vi "command data test.vi"() -> ()   [LabVIEW 2020]
panel:
  out "number":u32=24
  out "Array 2":string[](array[string])=["init\r\n", "runRange\r\n", "trackOn\r\n", "trackOff\r\n", "setLoad>1\r\n", "setMot>1\r\n", "setKp>1\r\n", "setKi>1\r\n", "setKd>1\r\n", "setR>1\r\n", "setG>1\r\n", "setB>1\r\n", "motOn\r\n", "motOff\r\n", "getVolts<1\r\n", "getBV<2\r\n", "getVal<1\r\n", "getKW<1\r\n", "getCarbon<1\r\n", "getAll<7\r\n", "getRes<1\r\n", "getDrop<1\r\n", "getCurrent<1\r\n", "off\r\n", "eoc\r\n"]
  out "Count":dbl=22.0
  in  "Array":string[](array[string])=["init", "runRange", "trackOn", "trackOff", "setLoad>1", "setMot>1", "setKp>1", "setKi>1", "setKd>1", "setR>1", "setG>1", "setB>1", "motOn", "motOff", "getVolts<1", "getBV<2", "getVal<1", "getKW<1", "getCarbon<1", "getAll<7", "getRes<1", "getDrop<1", "getCurrent<1", "off", "eoc"]
  in  "String":string="\"init\",\"runRange\", \"trackOn\",\"trackOff\",\n                    \"setLoad>1\",\"setMot>1\",\"setKp>1\",\"setKi>1\",\"setKd>1\",\"setR>1\",\"setG>1\",\"setB>1\",\n                    \"motOn\",\"motOff\",\n                    \"getVolts<1\", \"getBV<2\",\n                    \"getVal<1\",\"getKW<1\",\"getCarbon<1\",\"getAll<7\",\"getRes<1\",\"getDrop<1\",\"getCurrent<1\", \n                    \"off\",\"eoc\""
  out "read buffer":string="eoc\r\n"
  out "Device Name 2":string[](array[string])=["generator\r\n"]
  out "Num Dev 2":u32=1
  out "Device Address 2":refnum<visa-resource-name>[](array[refnum])=["ASRL28::INSTR"]
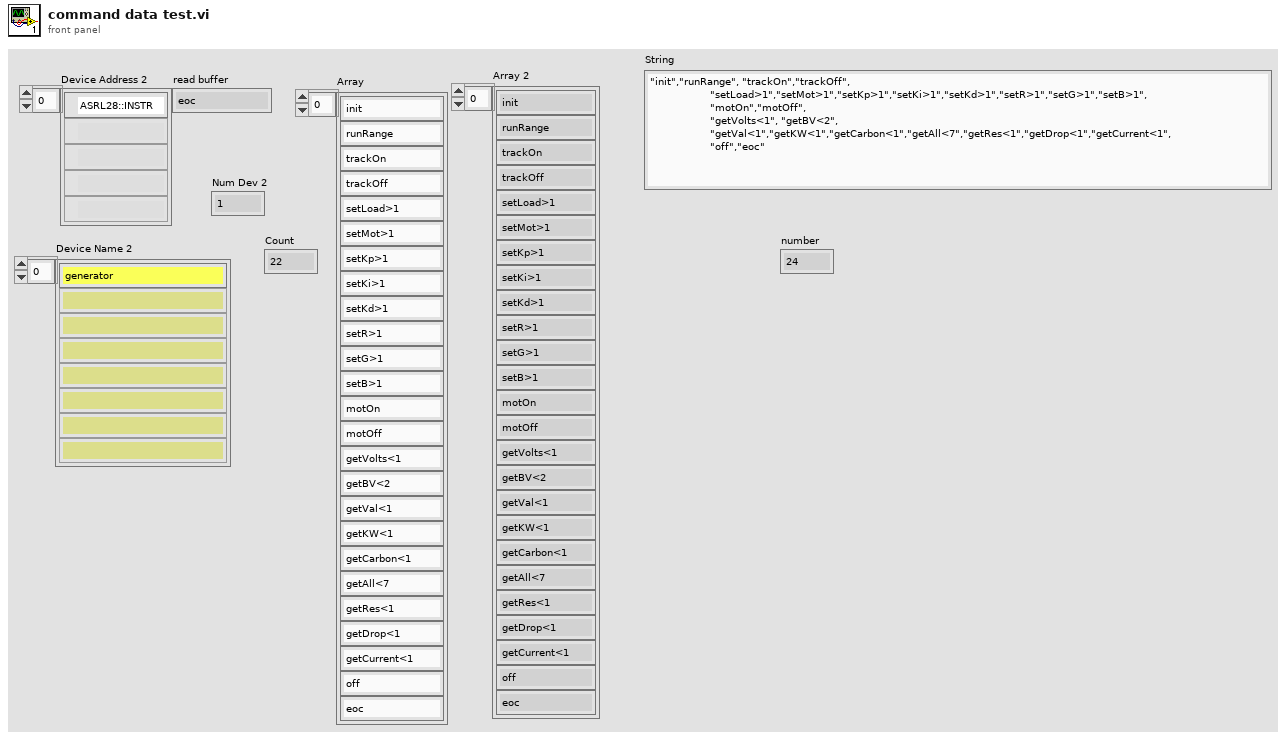
[diagram p1: front panel]
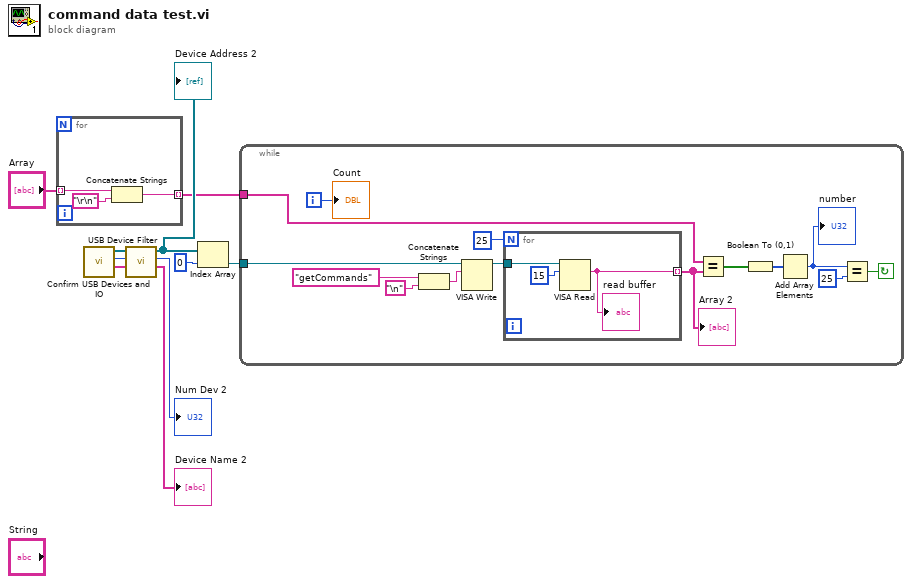
[diagram p0: block diagram]
diagram:
  n1 = for {
    tunnel: "Array" -> [w12] mode=indexing
    tunnel: [w11] -> w1 mode=indexing
    n2 = Concatenate Strings(w12, "\r\n") -> (w11:string)
  }
  n3 = call "Confirm USB Devices and IO.vi"() -> ("Device Name"=w10:string[], "Num Dev"=w9:u32, "Device Address"=w8:refnum<visa-resource-name>[])  [unwired: 9 in]
  n4 = call "USB Device Filter.vi"("Device Name"=w10, "Num Dev"=w9, "Device Address"=w8) -> ("Device Name 2"=→"Device Name 2":string[], "Num Dev 2"=→"Num Dev 2":u32, "Device Address 2"=w5:refnum<visa-resource-name>[])  [unwired: 6 in]
  "Device Address 2" <- w5
  n5 = Index Array(array=w5, index=0) -> (element=w3:refnum<visa-resource-name>)
  n6 = while {
    tunnel: w3 -> [w24]
    tunnel: w1 -> [w20]
    i -> [w17]
    stop <- w14 continue-if-true
    n7 = Concatenate Strings("getCommands", "\n") -> (w26:string)
    n8 = VISA Write(VISA resource name=w24, write buffer=w26) -> (VISA resource name out=w23:refnum<visa-resource-name>)  [unwired: 1 in, 2 out]
    n9 = for {
      N: 25 -> [_]
      tunnel: w23 -> [w29]
      tunnel: [w28] -> w21 mode=indexing
      n10 = VISA Read(VISA resource name=w29, byte count=u32 15) -> (read buffer=w28:string)  [unwired: 1 in, 3 out]
      "read buffer" <- w28
    }
    "Array 2" <- w21
    n11 = Equal?(x=w20, y=w21) -> (x = y?=w19:bool[])
    n12 = Boolean To (0,1)(Boolean=w19) -> (0, 1=w18:i16[])
    n13 = Add Array Elements(numeric array=w18) -> (sum=w16:i16)
    "number" <- w16
    n14 = Equal?(x=w16, y=i16 25) -> (x = y?=w14:bool)
    "Count" <- w17
  }
